vi "GetNumberOfPriorities.vi"(8 "error in":errorcluster, 11 "message ref in":refnum<class "CLM_PriorityLocalMessage.lvclass">) -> (0 "error out":errorcluster, 2 "number of priorities":i32, 3 "message ref out":refnum<class "CLM_PriorityLocalMessage.lvclass">)   [LabVIEW 2013, in "CLM_PriorityLocalMessage.lvclass"]
uses:
  CLM_PriorityLocalMessage.lvclass
  CLM_PriorityLocalMessage.lvclass/CLM_PriorityLocalMessage.ctl
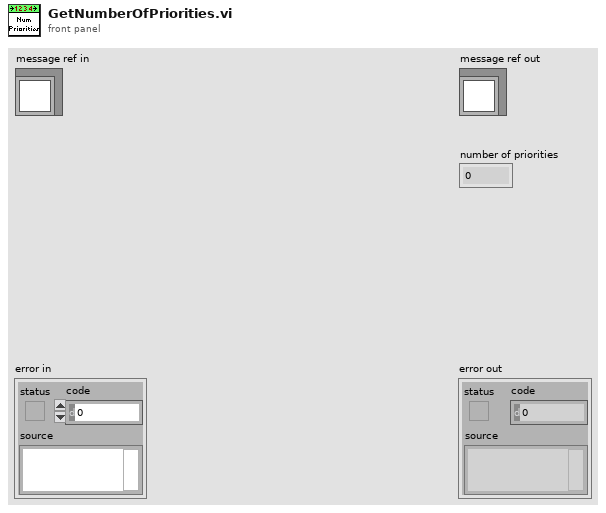
[diagram p1: front panel]
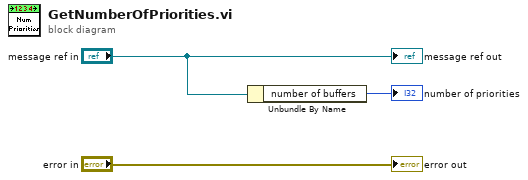
[diagram p0: block diagram]
diagram:
  n1 = Unbundle By Name("message ref in") -> ("number of buffers"=→"number of priorities":i32)
  "error out" <- "error in"
  "message ref out" <- "message ref in"
